vi "svl_Check for Overload.vi"(8 "error in (no error)":errorcluster, 9 "minimum input value (V)":dbl=-1.0 format="%.2f", 10 "maximum input value (V)":dbl=1.0 format="%.2f", 11 "signal [V]":waveform(dbl)={"t0"=timestamp(0 s since 1904-01-01), "dt"=0.0, "Y"=[]}) -> (0 "error out":errorcluster, 2 "overload":bool, 3 "dup signal [V]":waveform(dbl))   [LabVIEW 2017, in "SoundVib_Calibration.lvlib"]
uses:
  <vilib>/addons/Sound and Vibration/svt_Calibration/SoundVib_Calibration.lvlib
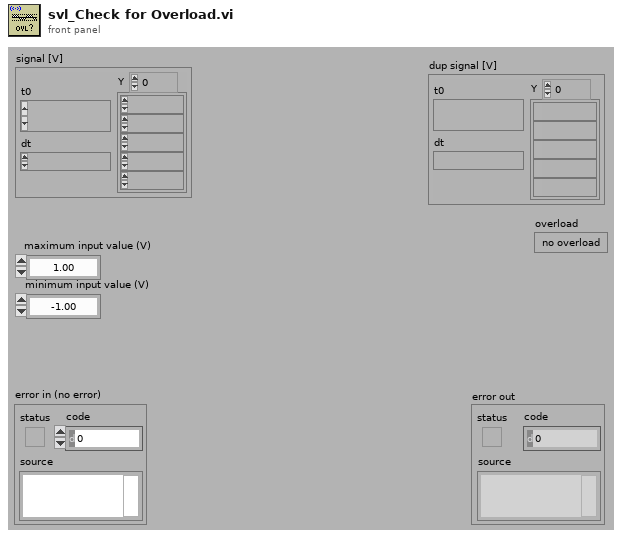
[diagram p1: front panel]
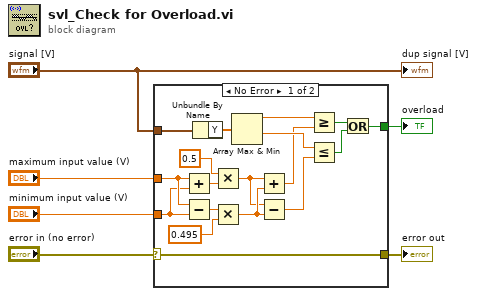
[diagram p0: block diagram]
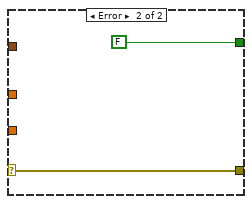
[diagram p2: hidden frame]
diagram:
  n1 = case shown="No Error" "error in (no error)" {
    selector: "error in (no error)" -> [w18 w25]
    tunnel: [w24 FALSE] -> w6
    tunnel: [w18 w25] -> w5
    tunnel: "signal [V]" -> [w17 _]
    tunnel: "maximum input value (V)" -> [w16 _]
    tunnel: "minimum input value (V)" -> [w15 _]
    frame No Error {
      n2 = Add(x=w16, y=w15) -> (x+y=w14:dbl)
      n3 = Subtract(x=w16, y=w15) -> (x-y=w12:dbl)
      n4 = Unbundle By Name(w17) -> ("Y"=w19:dbl[])
      n5 = Multiply(x=0.5, y=w14) -> (x*y=w8:dbl)
      n6 = Multiply(x=w12, y=0.495 ("x")) -> (x*y=w9:dbl)
      n7 = Array Max & Min(array=w19) -> (max value=w23:dbl, min value=w22:dbl)  [unwired: 2 out]
      n8 = Add(x=w8, y=w9) -> (x+y=w10:dbl)
      n9 = Subtract(x=w8, y=w9) -> (x-y=w7:dbl)
      n10 = Greater Or Equal?(x=w23, y=w10) -> (x >= y?=w21:bool)
      n11 = Less Or Equal?(x=w22, y=w7) -> (x <= y?=w20:bool)
      n12 = Or(x=w21, y=w20) -> (x .or. y?=w24:bool)
    }
    frame Error {
    }
  }
  "overload" <- w6
  "error out" <- w5
  "dup signal [V]" <- "signal [V]"
